vi "Ej_17_BCD_7_Segmentos.vi"() -> ()   [LabVIEW 2021]
panel:
  in  "stop":bool
  in  "Frecuencia":u32
  out "P1.2":bool
  out "P1.1.":bool
  out "A 3":bool
  out "B 3":bool
  out "G 3":bool
  out "D 3":bool
  out "C 3":bool
  out "E 3":bool
  out "F 3":bool
  out "F 2":bool
  out "E 2":bool
  out "C 2":bool
  out "D 2":bool
  out "G 2":bool
  out "B 2":bool
  out "A 2":bool
  in  "Stop":bool
  out "F":bool
  out "E":bool
  out "C":bool
  out "D":bool
  out "G":bool
  out "B":bool
  out "A":bool
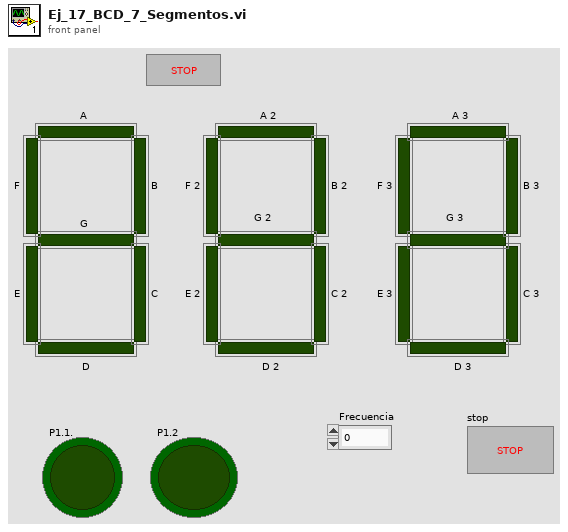
[diagram p1: front panel]
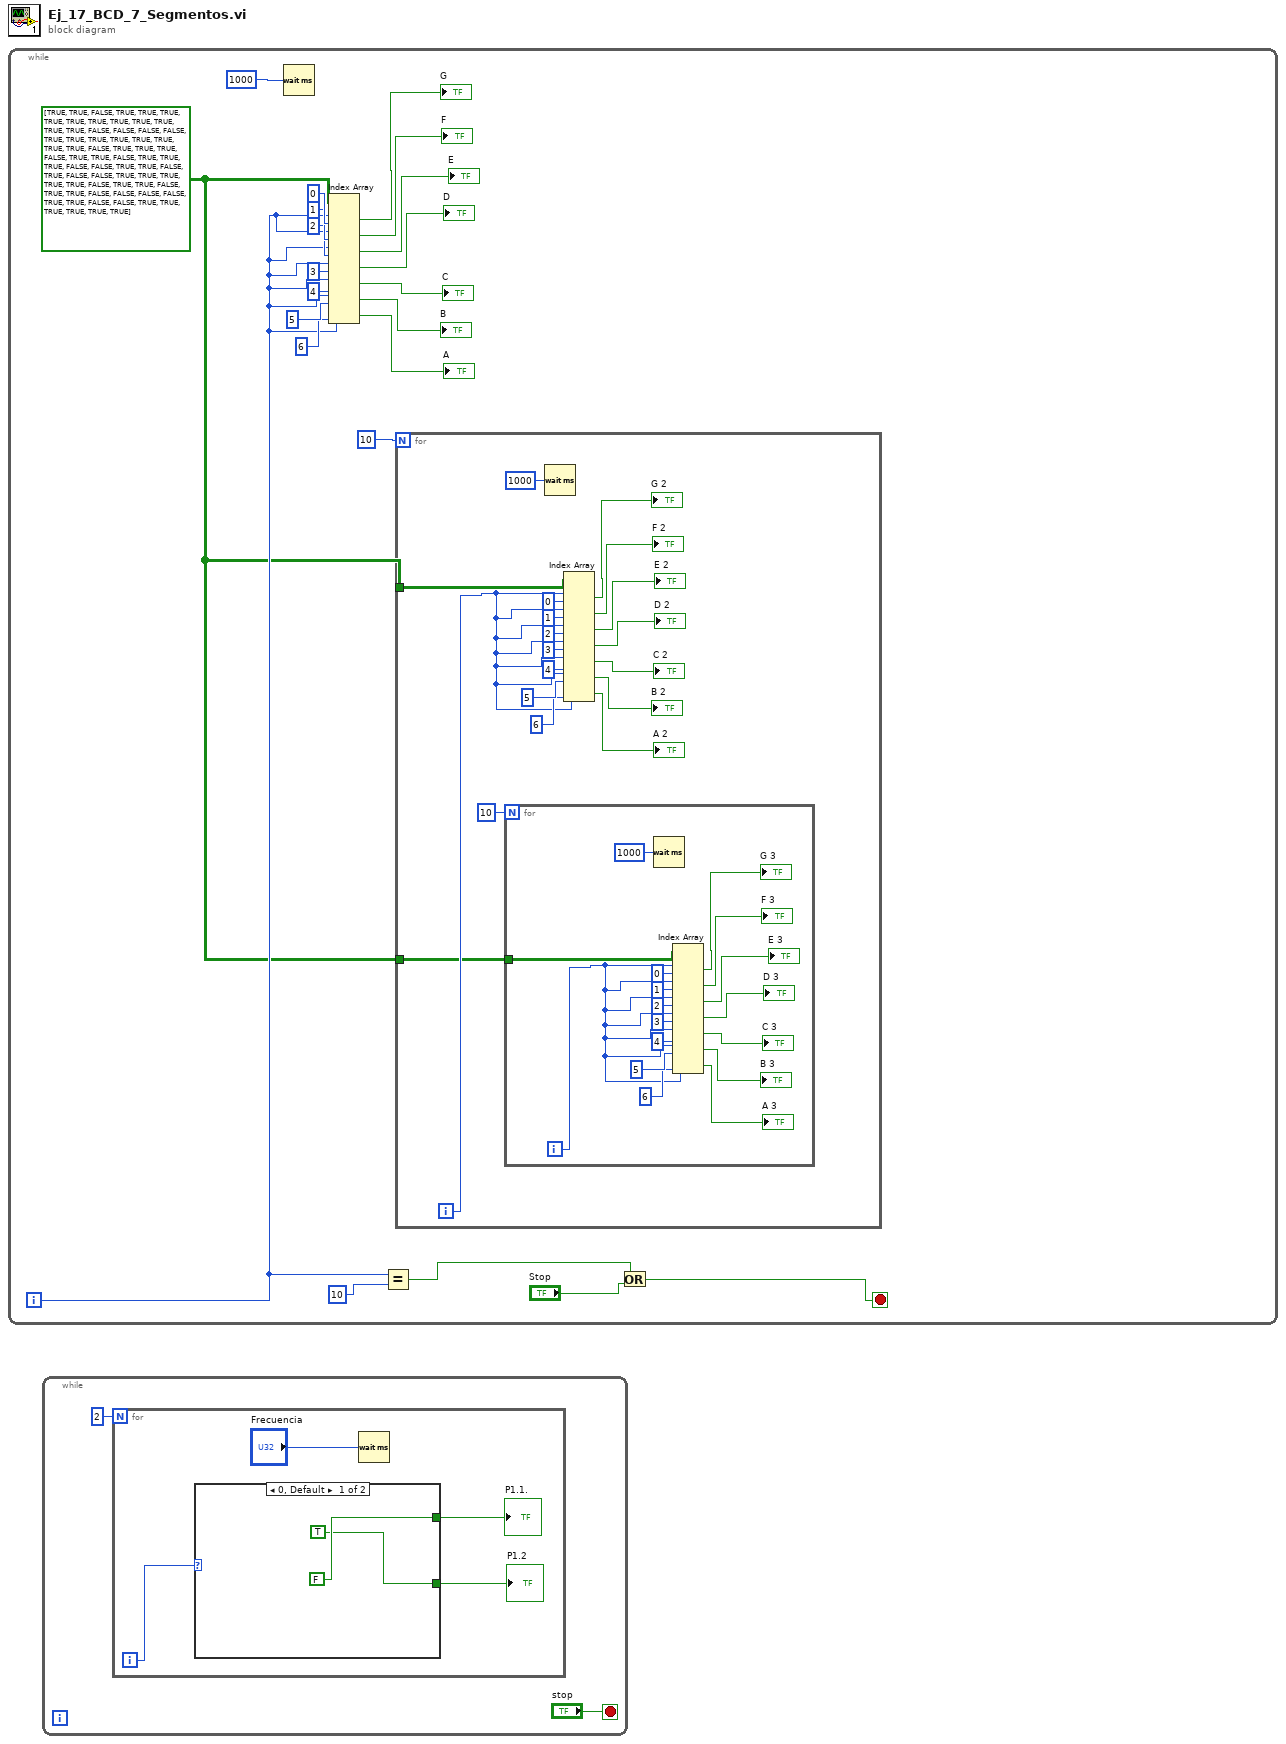
[diagram p0: block diagram]
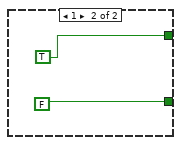
[diagram p2: hidden frame]
diagram:
  n1 = while {
    i -> [w3]
    stop <- w5 stop-if-true
    w1 = bool[][] [[TRUE, TRUE, FALSE, TRUE, TRUE, TRUE, TRUE], [TRUE, TRUE, TRUE, TRUE, TRUE, TRUE, TRUE], [FALSE, FALSE, FALSE, FALSE, TRUE, TRUE, TRUE], [TRUE, TRUE, TRUE, TRUE, TRUE, FALSE, TRUE], [TRUE, TRUE, FALSE, TRUE, TRUE, FALSE, TRUE], [TRUE, TRUE, FALSE, FALSE, TRUE, TRUE, FALSE], [TRUE, FALSE, FALSE, TRUE, TRUE, TRUE, TRUE], [TRUE, FALSE, TRUE, TRUE, FALSE, TRUE, TRUE], [FALSE, FALSE, FALSE, FALSE, TRUE, TRUE, FALSE], [FALSE, TRUE, TRUE, TRUE, TRUE, TRUE, TRUE]]
    n2 = Wait (ms)(milliseconds to wait=u32 1000 ("millisecond timer value")) -> ()  [unwired: 1 out]
    n3 = Index Array(array=w1, index (row) #1=w3, index (col) #1=0 ("disabled index (col)"), index (row) #2=w3, index (col) #2=1 ("disabled index (col)"), index (row) #3=w3, index (col) #3=2 ("disabled index (col)"), index (row) #4=w3, index (col) #4=3 ("disabled index (col)"), index (row) #5=w3, index (col) #5=4 ("disabled index (col)"), index (row) #6=w3, index (col) #6=5 ("disabled index (col)"), index (row) #7=w3, index (col) #7=6 ("index (col)")) -> (element #1=→"G":bool, element #2=→"F":bool, element #3=→"E":bool, element #4=→"D":bool, element #5=→"C":bool, element #6=→"B":bool, element #7=→"A":bool)
    n4 = Equal?(x=w3, y=10) -> (x = y?=w6:bool)
    n5 = for {
      N: 10 -> [_]
      tunnel: w1 -> [w27]
      tunnel: w1 -> [w23]
      i -> [w26]
      n6 = for {
        N: 10 -> [_]
        tunnel: w23 -> [w44]
        i -> [w43]
        n7 = Wait (ms)(milliseconds to wait=u32 1000) -> ()  [unwired: 1 out]
        n8 = Index Array(array=w44, index (row) #1=w43, index (col) #1=0 ("disabled index (col)"), index (row) #2=w43, index (col) #2=1 ("disabled index (col)"), index (row) #3=w43, index (col) #3=2 ("disabled index (col)"), index (row) #4=w43, index (col) #4=3 ("disabled index (col)"), index (row) #5=w43, index (col) #5=4 ("disabled index (col)"), index (row) #6=w43, index (col) #6=5 ("disabled index (col)"), index (row) #7=w43, index (col) #7=6 ("index (col)")) -> (element #1=→"G 3":bool, element #2=→"F 3":bool, element #3=→"E 3":bool, element #4=→"D 3":bool, element #5=→"C 3":bool, element #6=→"B 3":bool, element #7=→"A 3":bool)
      }
      n9 = Wait (ms)(milliseconds to wait=u32 1000) -> ()  [unwired: 1 out]
      n10 = Index Array(array=w27, index (row) #1=w26, index (col) #1=0 ("disabled index (col)"), index (row) #2=w26, index (col) #2=1 ("disabled index (col)"), index (row) #3=w26, index (col) #3=2 ("disabled index (col)"), index (row) #4=w26, index (col) #4=3 ("disabled index (col)"), index (row) #5=w26, index (col) #5=4 ("disabled index (col)"), index (row) #6=w26, index (col) #6=5 ("disabled index (col)"), index (row) #7=w26, index (col) #7=6 ("index (col)")) -> (element #1=→"G 2":bool, element #2=→"F 2":bool, element #3=→"E 2":bool, element #4=→"D 2":bool, element #5=→"C 2":bool, element #6=→"B 2":bool, element #7=→"A 2":bool)
    }
    n11 = Or(x=w6, y="Stop") -> (x .or. y?=w5:bool)
  }
  n12 = while {
    stop <- "stop" stop-if-true
    n13 = for {
      N: 2 -> [_]
      i -> [w61]
      n14 = case shown="0, Default" w61 {
        tunnel: [FALSE TRUE] -> w63
        tunnel: [TRUE FALSE] -> w62
        frame 0, Default {
        }
        frame 1 {
        }
      }
      "P1.1." <- w63
      "P1.2" <- w62
      n15 = Wait (ms)(milliseconds to wait="Frecuencia") -> ()  [unwired: 1 out]
    }
  }
